vi "ROI grp-Event Case-Table value change.vi"(8 "error in (no error)":errorcluster, 10 "NewVal":string[][](array[string]), 11 "OldVal":string[][](array[string])) -> (0 "error out":errorcluster)   [LabVIEW 2013]
uses:
  Typedefs/Get-Set-Clear Control.ctl
  Experiment header interface/Typedefs/Save-Load-Save as-Load last enum.ctl
  Globals/gl_ROI grp window globals.vi
panel:
  out "NewVal out":string[][](array[string])
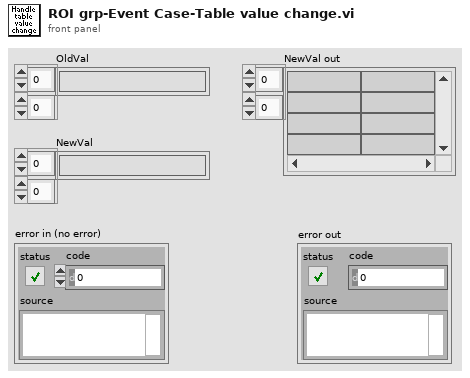
[diagram p1: front panel]
types:
  T1 = typedef "ROI grp-window ctrl refs.ctl" = cluster{"This VI":refnum<vi>, "Pane":refnum<vi>, "Table":refnum<vi>}
  T2 = typedef "Save-Load-Save as-Load last enum.ctl" = enum16{"Save file", "Save file as", "Load file", "Load last file"}
  T3 = typedef "Get-Set-Clear Control.ctl" = enum16{"Get", "Set", "Clear"}
  T4 = typedef "ROI group info cluster.ctl" = cluster{"Group name":string, "# ROI in group":i32, "ROI numbers in group":i32[], "Group region specifier cluster":T5}
  T5 = typedef "ROI Descriptor" = cluster{"Global Rectangle":i32[], "Contours":cluster{"ID":enum32{"External", "Internal"}, "Type":u32, "Coordinates":i32[]}[]}
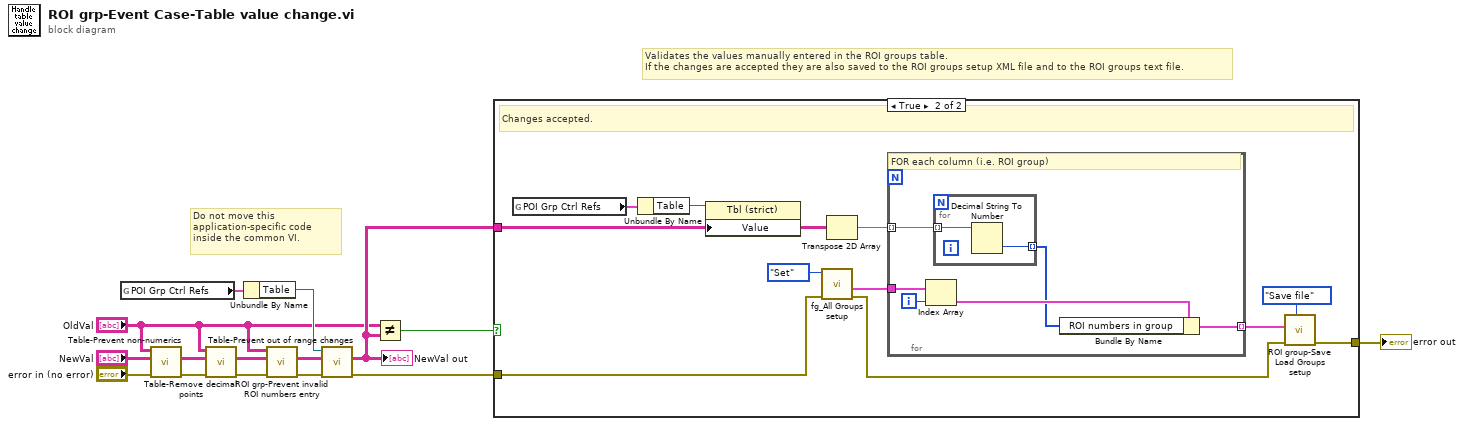
[diagram p0: block diagram]
diagram:
  # "Validates the values manually entered in the ROI groups table.\nIf the changes are accepted they are also saved to the ROI groups setup XML file and to the ROI groups text file."
  # "Do not move this application-specific code inside the common VI."
  n1 = global read "gl_ROI grp window globals.vi" "POI Grp Ctrl Refs"() -> (w12:T1)
  n2 = call "Table-Prevent non-numerics.vi"("error in (no error)"="error in (no error)", "NewVal in"="NewVal", "OldVal"="OldVal") -> ("error out"=w14:errorcluster, "Val out"=w15:string[][])  [unwired: 6 in, 1 out]
  n3 = call "Table-Remove decimal points.vi"("error in (no error)"=w14, "NewVal"=w15, "OldVal"="OldVal") -> ("error out"=w9:errorcluster, "NewVal out"=w7:string[][])  [unwired: 7 in]
  n4 = Unbundle By Name(w12) -> ("Table"=w13:refnum<vi>)
  n5 = call "ROI grp-Prevent invalid ROI numbers entry.vi"("error in (no error)"=w9, "NewVal in"=w7, "OldVal"="OldVal") -> ("error out"=w8:errorcluster, "Val out"=w6:string[][])  [unwired: 6 in, 1 out]
  n6 = call "Table-Prevent out of range changes.vi"("error in (no error)"=w8, "Table Value in"=w6, "Table ref in"=w13) -> ("error out"=w5:errorcluster, "Table Value out"=w3:string[][])  [unwired: 6 in, 1 out]
  "NewVal out" <- w3
  n7 = Not Equal?(x="OldVal", y=w3) -> (x != y?=w1:bool)
  n8 = case shown="True" w1 {
    tunnel: w5 -> [w16 w20]
    tunnel: [w16 w18] -> w4
    tunnel: w3 -> [_ w17]
    frame False {
      # "Changes rejected."
    }
    frame True {
      # "Changes accepted."
      n9 = global read "gl_ROI grp window globals.vi" "POI Grp Ctrl Refs"() -> (w27:T1)
      n10 = Unbundle By Name(w27) -> ("Table"=w26:refnum<vi>)
      n11 = property class="Tbl (strict)"(reference=w26, "Value"=w17) -> ()  [unwired: 1 in, 2 out]
      n12 = call "fg_All Groups setup.vi"("error in (no error)"=w20, "Function"=Get-Set-Clear_Control."Set") -> ("error out"=w19:errorcluster, "Groups setup out"=w24:T4[])  [unwired: 8 in]
      n13 = Transpose 2D Array(2D array=w17) -> (transposed array=w21:string[][])
      n14 = for {
        tunnel: w24 -> [w33]
        tunnel: w21 -> [w29] mode=indexing
        tunnel: [w30] -> w22 mode=indexing
        i -> [w32]
        # "FOR each column (i.e. ROI group)"
        n15 = Index Array(array=w33, index=w32) -> (element=w31:T4)
        n16 = for {
          tunnel: w29 -> [w35] mode=indexing
          tunnel: [w34] -> w28 mode=indexing
          n17 = Decimal String To Number(string=w35) -> (number=w34:i32)  [unwired: 2 in, 1 out]
        }
        n18 = Bundle By Name(cluster=w31, "ROI numbers in group"=w28) -> (w30:T4)
      }
      n19 = call "ROI group-Save Load Groups setup.vi"("error in (no error)"=w19, "Function"=Save-Load-Save_as-Load_last_enum."Save file", "Groups setup to save"=w22) -> ("error out"=w18:errorcluster)  [unwired: 7 in, 1 out]
    }
  }
  "error out" <- w4
